vi "GetLocalComputerName.vi"() -> (2 "Name":string, 3 "Full Name":string)   [LabVIEW 2013]
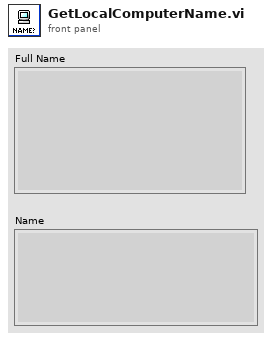
[diagram p1: front panel]
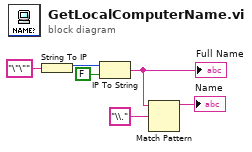
[diagram p0: block diagram]
diagram:
  n1 = String To IP(1:"\"\"" ("name")) -> (0:w5:u32)
  n2 = IP To String(1:FALSE ("dot notation? (F)"), 2:w5) -> (0:w1:string)
  "Full Name" <- w1
  n3 = Match Pattern(string=w1, regular expression="\\.") -> (before substring=→"Name":string)  [unwired: 1 in, 3 out]
